vi "Write Region.vi"(8 "error in (no error)":errorcluster, 10 "Region":T1, 11 "AWS Core in":refnum<class "NI_AWS_Core.lvclass">) -> (0 "error out":errorcluster, 3 "AWS Core out":refnum<class "NI_AWS_Core.lvclass">)   [LabVIEW 2015, in "NI_AWS_Core.lvclass"]
uses:
  NI_AWS_Core.lvclass
  Region.ctl
  NI_AWS_Core.lvclass/NI_AWS_Core.ctl
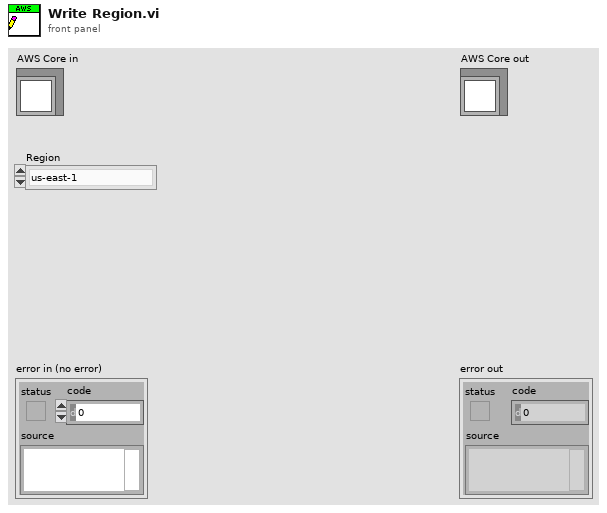
[diagram p1: front panel]
types:
  T1 = typedef "NI_AWS_Core.lvclass/Region.ctl" = enum16{"us-east-1", "us-east-2", "us-west-1", "us-west-2", "ap-northeast-1", "ap-northeast-2", "ap-southeast-1", "ap-southeast-2", "ca-central-1", "eu-central-1", "eu-west-1", "eu-west-2", "sa-east-1"}
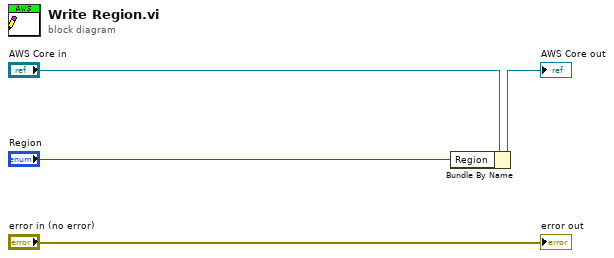
[diagram p0: block diagram]
diagram:
  n1 = Bundle By Name(cluster="AWS Core in", "Region"="Region") -> (→"AWS Core out":refnum<class "NI_AWS_Core.lvclass">)
  "error out" <- "error in (no error)"
